vi "Calculate Average Center.vi"(9 "Hexaboard Version":i32, 10 "Position":i32, 11 "Gantry Fiducials":dbl[](array[numeric])) -> (1 "Sensor ID Location":dbl[](array[numeric]), 2 "CH1 Location":dbl[](array[numeric]), 3 "XYZTheta":dbl[](array[numeric]))   [LabVIEW 2021, in "Component Tray.lvclass"]
uses:
  Component Tray.lvclass
  <vilib>/Analysis/baseanly.llb/Mean (DBL).vi
  <vilib>/Analysis/NI_AALBase.lvlib
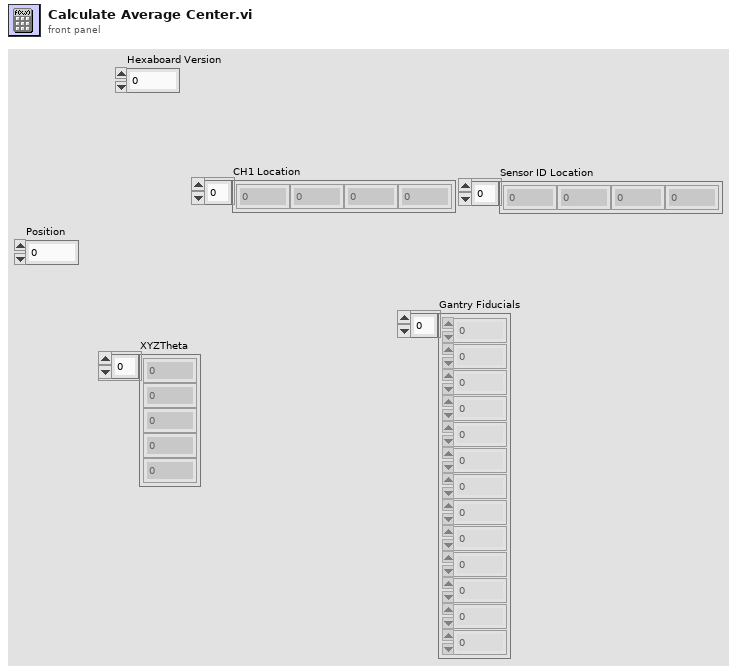
[diagram p1: front panel]
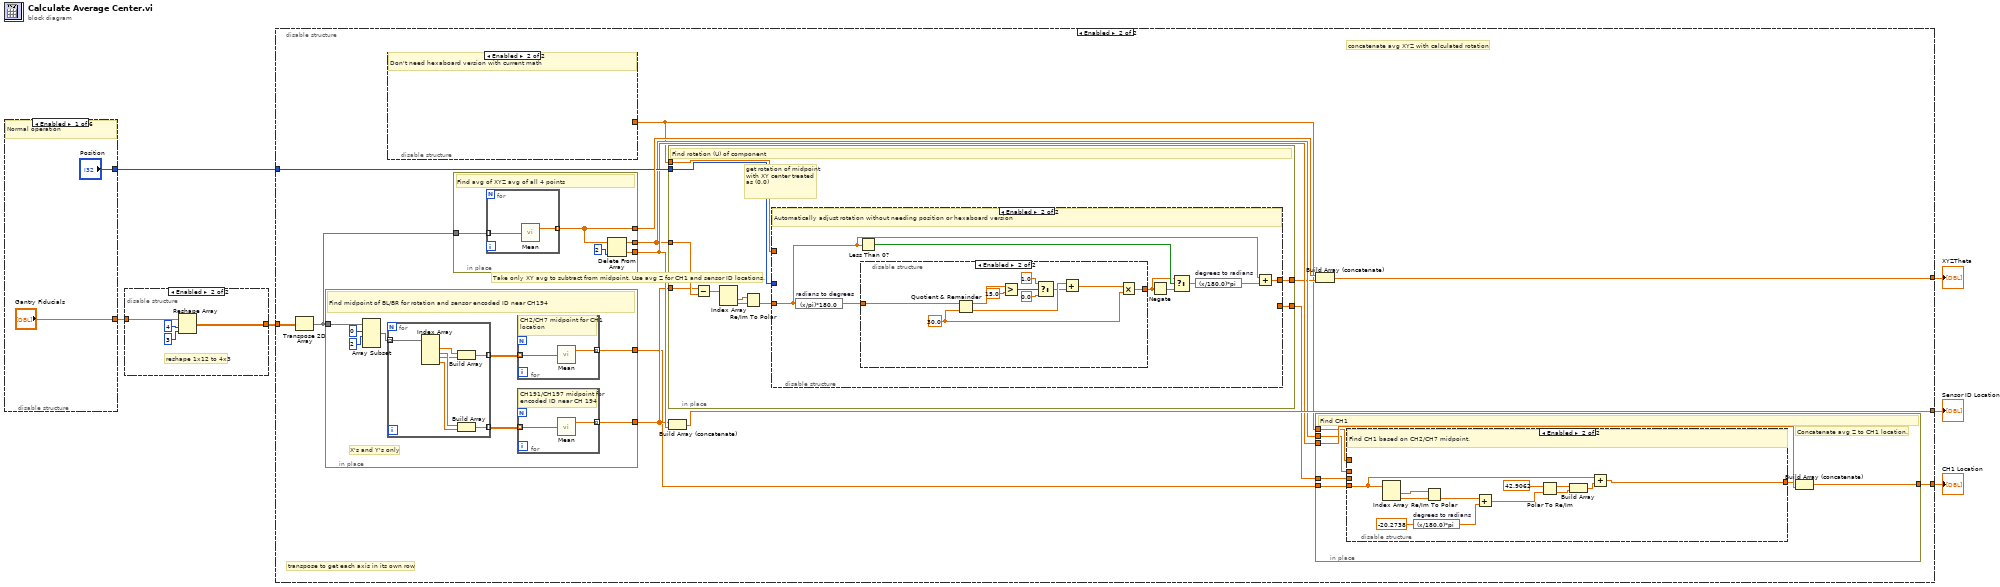
[diagram p0: block diagram]
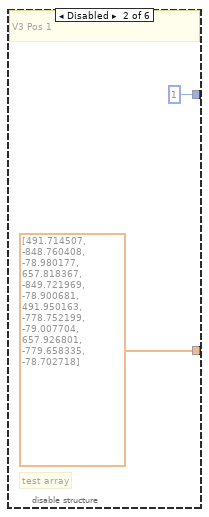
[diagram p2: hidden frame]
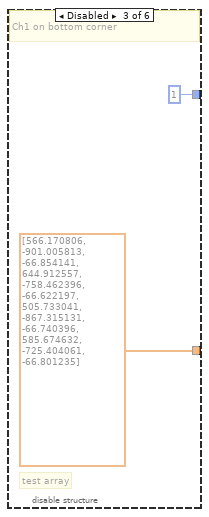
[diagram p3: hidden frame]
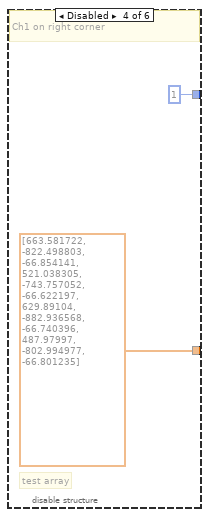
[diagram p4: hidden frame]
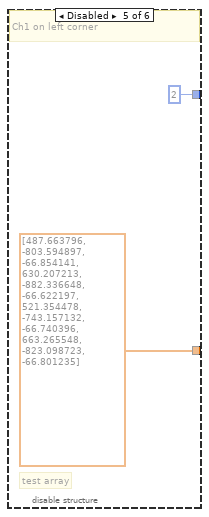
[diagram p5: hidden frame]
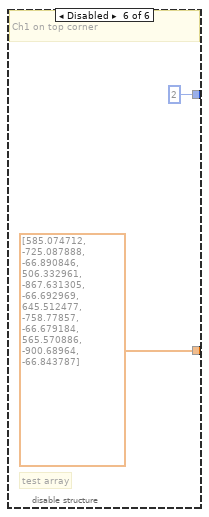
[diagram p6: hidden frame]
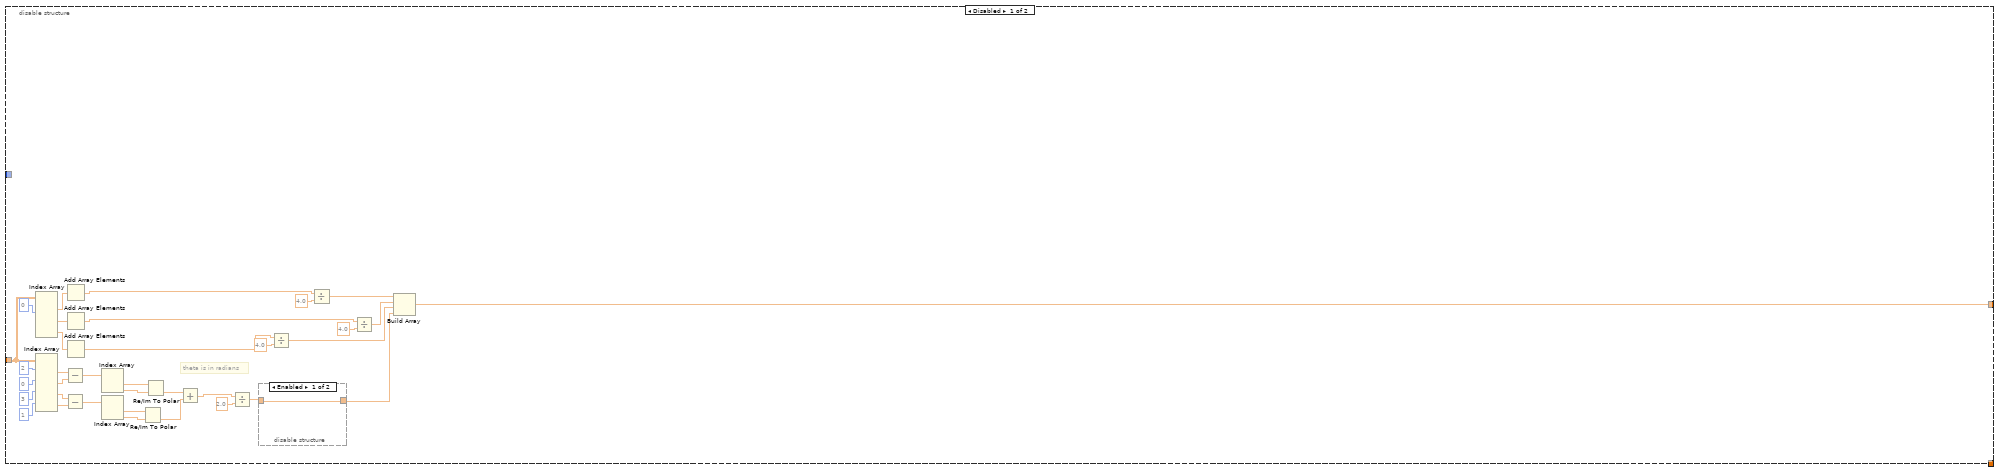
[diagram p7: hidden frame]
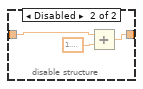
[diagram p8: hidden frame]
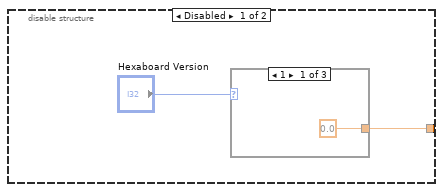
[diagram p9: hidden frame]
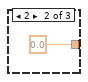
[diagram p10: hidden frame]
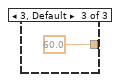
[diagram p11: hidden frame]
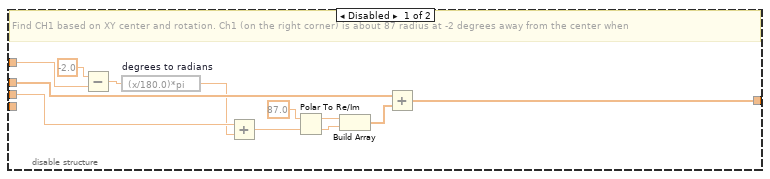
[diagram p12: hidden frame]
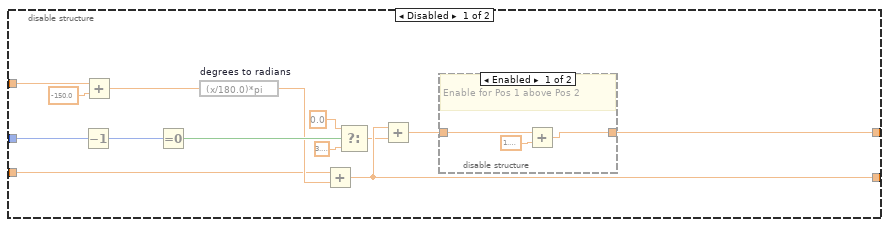
[diagram p13: hidden frame]
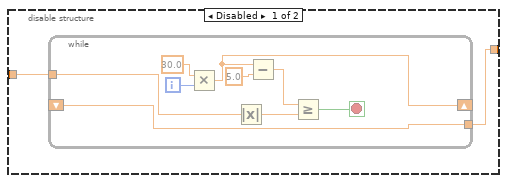
[diagram p15: hidden frame]
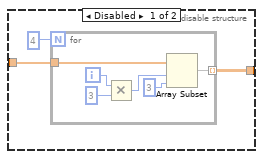
[diagram p16: hidden frame]
diagram:
  n1 = disable-structure shown="Enabled" {
    disable-tunnel: ["Gantry Fiducials" dbl[] [491.714507, -848.760408, -78.980177, 657.818367, -849.721969, -78.900681, 491.950163, -778.752199, -79.007704, 657.926801, -779.658335, -78.702718] dbl[] [566.170806, -901.005813, -66.854141, 644.912557, -758.462396, -66.622197, 505.733041, -867.315131, -66.740396, 585.674632, -725.404061, -66.801235] dbl[] [663.581722, -822.498803, -66.854141, 521.038305, -743.757052, -66.622197, 629.89104, -882.936568, -66.740396, 487.97997, -802.994977, -66.801235] dbl[] [487.663796, -803.594897, -66.854141, 630.207213, -882.336648, -66.622197, 521.354478, -743.157132, -66.740396, 663.265548, -823.098723, -66.801235] dbl[] [585.074712, -725.087888, -66.890846, 506.332961, -867.631305, -66.692969, 645.512477, -758.77857, -66.679184, 565.570886, -900.68964, -66.843787]] -> w5
    disable-tunnel: ["Position" 1 ("Position") 1 ("Position") 1 ("Position") 2 ("Position") 2 ("Position")] -> w1
    frame Enabled {
      # "Normal operation"
    }
    frame Disabled {
      # "test array"
      # "V3 Pos 1"
    }
    frame Disabled {
      # "test array"
      # "Ch1 on bottom corner"
    }
    frame Disabled {
      # "test array"
      # "Ch1 on right corner"
    }
    frame Disabled {
      # "test array"
      # "Ch1 on left corner"
    }
    frame Disabled {
      # "test array"
      # "Ch1 on top corner"
    }
  }
  n2 = disable-structure shown="Enabled" {
    disable-tunnel: w5 -> [w21 w31]
    disable-tunnel: [w20 w28] -> w2
    frame Disabled {
      n3 = for {
        N: 4 -> [_]
        tunnel: w21 -> [w23]
        tunnel: [w22] -> w20 mode=indexing
        i -> [w27]
        n4 = Multiply(x=w27, y=3) -> (x*y=w25:i32)
        n5 = Array Subset(array=w23, index=w25, length=3) -> (w22:dbl[])
      }
    }
    frame Enabled {
      # "reshape 1x12 to 4x3"
      n6 = Reshape Array(w31, 4 ("dimension size"), 3 ("dimension size")) -> (w28:dbl[][])
    }
  }
  n7 = disable-structure shown="Enabled" {
    disable-tunnel: [w36 w83] -> w6
    disable-tunnel: w2 -> [w35 w84]
    disable-tunnel: [_ w79] -> w4
    disable-tunnel: [_ w82] -> w3
    disable-tunnel: w1 -> [_ w78]
    frame Disabled {
      # "theta is in radians"
      n8 = Index Array(array=w35, index (col) #1=0 ("disabled index (col)")) -> (element #1=w65:dbl[], element #2=w64:dbl[], element #3=w34:dbl[])  [unwired: 5 in]
      n9 = Index Array(array=w35, index (row) #1=2 ("index (row)"), index (row) #2=0 ("index (row)"), index (row) #3=3 ("index (row)"), index (row) #4=1 ("index (row)")) -> (element #1=w49:dbl[], element #2=w48:dbl[], element #3=w47:dbl[], element #4=w46:dbl[])  [unwired: 4 in]
      n10 = Subtract(x=w49, y=w48) -> (x-y=w59:dbl[])
      n11 = Subtract(x=w47, y=w46) -> (x-y=w58:dbl[])
      n12 = Add Array Elements(numeric array=w65) -> (sum=w63:dbl)
      n13 = Add Array Elements(numeric array=w64) -> (sum=w62:dbl)
      n14 = Add Array Elements(numeric array=w34) -> (sum=w40:dbl)
      n15 = Index Array(array=w59) -> (element #1=w57:dbl, element #2=w56:dbl)  [unwired: 2 in]
      n16 = Index Array(array=w58) -> (element #1=w55:dbl, element #2=w54:dbl)  [unwired: 2 in]
      n17 = Re/Im To Polar(2:w54, 3:w55) -> (0:w52:dbl)  [unwired: 1 out]
      n18 = Re/Im To Polar(2:w56, 3:w57) -> (0:w53:dbl)  [unwired: 1 out]
      n19 = Add(x=w53, y=w52) -> (x+y=w51:dbl)
      n20 = Divide(x=w51, y=2.0) -> (x/y=w33:dbl)
      n21 = disable-structure shown="Enabled" {
        disable-tunnel: w33 -> [w67 w69]
        disable-tunnel: [w67 w68] -> w32
        frame Enabled {
        }
        frame Disabled {
          n22 = Add(x=w69, y=1.5707963267948966) -> (x+y=w68:dbl)
        }
      }
      n23 = Divide(x=w40, y=4.0) -> (x/y=w37:dbl)
      n24 = Divide(x=w63, y=4.0) -> (x/y=w39:dbl)
      n25 = Divide(x=w62, y=4.0) -> (x/y=w38:dbl)
      n26 = Build Array(w39, w38, w37, w32) -> (w36:dbl[])
    }
    frame Enabled {
      # "concatenate avg XYZ with calculated rotation"
      # "Take only XY avg to subtract from midpoint. Use avg Z for CH1 and sensor ID locations."
      # "transpose to get each axis in its own row"
      n27 = Transpose 2D Array(2D array=w84) -> (transposed array=w80:dbl[][])
      n28 = in-place {
        in-place-border: w80 -> [w186]
        in-place-border: [w181] -> w76
        in-place-border: [w179] -> w71
        # "X's and Y's only"
        # "Find midpoint of BL/BR for rotation and sensor encoded ID near CH194"
        n29 = Array Subset(array=w186, index (row)=0 ("index"), length (row)=2 ("length")) -> (w183:dbl[][])  [unwired: 2 in]
        n30 = for {
          tunnel: w183 -> [w197] mode=indexing
          tunnel: [w194] -> w182 mode=indexing
          tunnel: [w191] -> w180 mode=indexing
          n31 = Index Array(array=w197) -> (element #1=w193:dbl, element #2=w196:dbl, element #3=w192:dbl, element #4=w195:dbl)  [unwired: 4 in]
          n32 = Build Array(w193, w192) -> (w191:dbl[])
          n33 = Build Array(w196, w195) -> (w194:dbl[])
        }
        n34 = for {
          tunnel: w180 -> [w187] mode=indexing
          tunnel: [w188] -> w179 mode=indexing
          # "CH2/CH7 midpoint for CH1 location"
          n35 = call-poly <vilib>:"Mean.vi"("X"=w187) -> ("mean"=w188:dbl)  [unwired: 1 out]
        }
        n36 = for {
          tunnel: [w189] -> w181 mode=indexing
          tunnel: w182 -> [w190] mode=indexing
          # "CH191/CH197 midpoint for encoded ID near CH 194"
          n37 = call-poly <vilib>:"Mean.vi"("X"=w190) -> ("mean"=w189:dbl)  [unwired: 1 out]
        }
      }
      n38 = disable-structure shown="Enabled" {
        disable-tunnel: [w85 _] -> w72
        frame Disabled {
          n39 = case shown="1" "Hexaboard Version" {
            tunnel: [0.0 0.0 60.0] -> w85
            frame 1 {
            }
            frame 2 {
            }
            frame 3, Default {
            }
          }
        }
        frame Enabled {
          # "Don't need hexaboard version with current math"
        }
      }
      n40 = in-place {
        in-place-border: w80 -> [w202]
        in-place-border: [w201] -> w81
        in-place-border: [w199] -> w77
        in-place-border: [w198] -> w74
        # "Find avg of XYZ avg of all 4 points"
        n41 = for {
          tunnel: [w204] -> w201 mode=indexing
          tunnel: w202 -> [w203] mode=indexing
          n42 = call-poly <vilib>:"Mean.vi"("X"=w203) -> ("mean"=w204:dbl)  [unwired: 1 out]
        }
        n43 = Delete From Array(array=w201, index=2) -> (deleted portion=w199:dbl, array with subset deleted=w198:dbl[])  [unwired: 1 in]
      }
      n44 = in-place {
        in-place-border: w74 -> [w127]
        in-place-border: w76 -> [w126]
        in-place-border: [w124] -> w75
        in-place-border: w78 -> [w125]
        in-place-border: [w123] -> w73
        in-place-border: w72 -> [w122]
        # "get rotation of midpoint with XY center treated as (0,0)"
        # "Find rotation (U) of component"
        n45 = Subtract(x=w126, y=w127) -> (x-y=w128:dbl[])
        n46 = Index Array(array=w128) -> (element #1=w129:dbl, element #2=w130:dbl)  [unwired: 2 in]
        n47 = Re/Im To Polar(2:w130, 3:w129) -> (0:w121:dbl)  [unwired: 1 out]
        n48 = disable-structure shown="Enabled" {
          disable-tunnel: w125 -> [w144 _]
          disable-tunnel: [w139 _] -> w124
          disable-tunnel: [w136 w153] -> w123
          disable-tunnel: w122 -> [w133 _]
          disable-tunnel: w121 -> [w131 w154]
          frame Disabled {
            n49 = Decrement(x=w144) -> (x-1=w142:i32)
            n50 = Add(x=w133, y=-150.0) -> (x+y=w132:dbl)
            n51 = Equal To 0?(x=w142) -> (x = 0?=w143:bool)
            n52 = expression code="(x/180.0)*pi" "degrees to radians"(w132) -> (w135:dbl)
            n53 = Add(x=w131, y=w135) -> (x+y=w139:dbl)
            n54 = Select(t=0.0, s=w143, f=3.141592653589793) -> (s? t:f=w138:dbl)
            n55 = Add(x=w139, y=w138) -> (x+y=w137:dbl)
            n56 = disable-structure shown="Enabled" {
              disable-tunnel: [w147 w148] -> w136
              disable-tunnel: w137 -> [w146 w148]
              frame Enabled {
                # "Enable for Pos 1 above Pos 2"
                n57 = Add(x=w146, y=1.5707963267948966) -> (x+y=w147:dbl)
              }
              frame Disabled {
                # "Enable for Pos 1 left of Pos 2"
              }
            }
          }
          frame Enabled {
            # "Automatically adjust rotation without needing position or hexaboard version"
            n58 = expression code="(x/pi)*180.0" "radians to degrees"(w154) -> (w152:dbl)
            n59 = Less Than 0?(x=w154) -> (x < 0?=w155:bool)
            n60 = disable-structure shown="Enabled" {
              disable-tunnel: [w158 w168] -> w150
              disable-tunnel: w152 -> [w157 w171]
              frame Disabled {
                n61 = while {
                  tunnel: w157 -> [w165]
                  shift-right: [w162] -> _
                  shift-left: _ -> [w163]
                  tunnel: [w163] -> w158
                  i -> [w166]
                  stop <- w161 stop-if-true
                  n62 = Multiply(x=30.0 ("y"), y=w166) -> (x*y=w162:dbl)
                  n63 = Absolute Value(x=w165) -> (abs(x)=w160:dbl)
                  n64 = Subtract(x=w162, y=5.0) -> (x-y=w159:dbl)
                  n65 = Greater Or Equal?(x=w159, y=w160) -> (x >= y?=w161:bool)
                }
              }
              frame Enabled {
                w169 = 30.0 ("y")
                n66 = Quotient & Remainder(x=w171, y=w169) -> (x-y*floor(x/y)=w175:dbl, floor(x/y)=w178:dbl)
                n67 = Greater?(x=w175, y=15.0) -> (0:w176:bool)
                n68 = Select(t=1.0, s=w176, f=0.0) -> (s? t:f=w177:dbl)
                n69 = Add(x=w178, y=w177) -> (x+y=w170:dbl)
                n70 = Multiply(x=w170, y=w169) -> (x*y=w168:dbl)
              }
            }
            n71 = Negate(x=w150) -> (-x=w151:dbl)
            n72 = Select(t=w150, s=w155, f=w151) -> (s? t:f=w149:dbl)
            n73 = expression code="(x/180.0)*pi" "degrees to radians"(w149) -> (w156:dbl)
            n74 = Add(x=w154, y=w156) -> (x+y=w153:dbl)
          }
        }
      }
      n75 = Build Array (concatenate)(w76, w77) -> (w82:dbl[])
      n76 = Build Array (concatenate)(w81, w73) -> (w83:dbl[])
      n77 = in-place {
        in-place-border: w74 -> [w93]
        in-place-border: w75 -> [w96]
        in-place-border: w77 -> [w95]
        in-place-border: [w94] -> w79
        in-place-border: w72 -> [w91]
        in-place-border: w71 -> [w90]
        # "Concatenate avg Z to CH1 location."
        # "Find CH1"
        n78 = disable-structure shown="Enabled" {
          disable-tunnel: w96 -> [w108 _]
          disable-tunnel: w93 -> [w107 _]
          disable-tunnel: [w106 w115] -> w92
          disable-tunnel: w91 -> [w97 _]
          disable-tunnel: w90 -> [_ w114]
          frame Disabled {
            # "Find CH1 based on XY center and rotation. Ch1 (on the right corner) is about 87 radius at -2 degrees away from the center when"
            n79 = Subtract(x=-2.0, y=w97) -> (x-y=w98:dbl)
            n80 = expression code="(x/180.0)*pi" "degrees to radians"(w98) -> (w101:dbl)
            n81 = Add(x=w108, y=w101) -> (x+y=w100:dbl)
            n82 = Polar To Re/Im(2:w100, 3:87.0 ("r")) -> (0:w103:dbl, 1:w104:dbl)
            n83 = Build Array(w104, w103) -> (w102:dbl[])
            n84 = Add(x=w107, y=w102) -> (x+y=w106:dbl[])
          }
          frame Enabled {
            # "Find CH1 based on CH2/CH7 midpoint."
            n85 = Index Array(array=w114) -> (element #1=w113:dbl, element #2=w112:dbl)  [unwired: 2 in]
            n86 = expression code="(x/180.0)*pi" "degrees to radians"(-20.2738) -> (w110:dbl)
            n87 = Re/Im To Polar(2:w112, 3:w113) -> (0:w111:dbl)  [unwired: 1 out]
            n88 = Add(x=w111, y=w110) -> (x+y=w109:dbl)
            n89 = Polar To Re/Im(2:w109, 3:42.9062 ("r")) -> (0:w117:dbl, 1:w118:dbl)
            n90 = Build Array(w118, w117) -> (w116:dbl[])
            n91 = Add(x=w114, y=w116) -> (x+y=w115:dbl[])
          }
        }
        n92 = Build Array (concatenate)(w92, w95) -> (w94:dbl[])
      }
    }
  }
  "XYZTheta" <- w6
  "CH1 Location" <- w4
  "Sensor ID Location" <- w3
